vi "Get Bucket Location.vi"(8 "error in (no error)":errorcluster, 9 "Bucket":string) -> (0 "error out":errorcluster, 3 "Region":T1)   [LabVIEW 2015, in "LV Interface for Amazon S3.lvlib"]
doc: "This operation <B>returns</B> a <B>bucket's Region</B>. You set the bucket's Region using the Region request parameter in a PUT Bucket request. To use this implementation of the operation, <B>you must be the bucket Owner</B>."
uses:
  LV Interface for Amazon S3.lvlib
  Typedefs/AMZ_S3_LocationConstraint.ctl
  XML Parser/XML Parser.lvlib
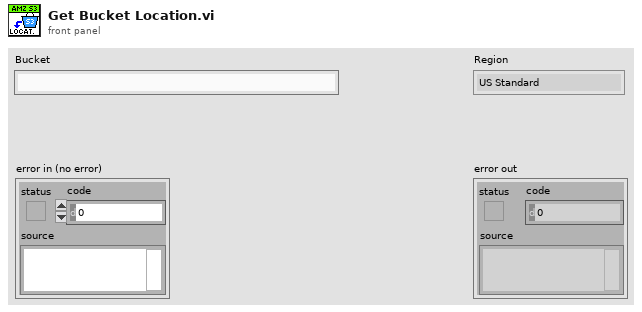
[diagram p1: front panel]
types:
  T1 = typedef "LV Interface for Amazon S3.lvlib/AMZ_S3_LocationConstraint.ctl" = enum16{"US Standard", "us-east-2", "us-west-1", "us-west-2", "ap-northeast-1", "ap-northeast-2", "ap-southeast-1", "ap-southeast-2", "ca-central-1", "eu-central-1", "eu-west-1", "eu-west-2", "sa-east-1"}
  T2 = typedef "LV Interface for Amazon S3.lvlib/AMZ_S3_Call Results.ctl" = enum16{"Success", "UndefinedError", "AccessDenied", "AccountProblem", "AmbiguousGrantByEmailAddress", "BadDigest", "BucketAlreadyExists", "BucketAlreadyOwnedByYou", "BucketNotEmpty", "CredentialsNotSupported", "CrossLocationLoggingProhibited", "EntityTooSmall", "EntityTooLarge", "ExpiredToken", "IllegalVersioningConfigurationException", "IncompleteBody", "IncorrectNumberOfFilesInPostRequest", "InlineDataTooLarge", "InternalError", "InvalidAccessKeyId", "InvalidAddressingHeader", "InvalidArgument", "InvalidBucketName", "InvalidDigest", "InvalidLocationConstraint", "InvalidPart", "InvalidPartOrder", "InvalidPayer", "InvalidPolicyDocument", "InvalidRange", "InvalidSecurity", "InvalidSOAPRequest", "InvalidStorageClass", "InvalidTargetBucketForLogging", "InvalidToken", "InvalidURI", "KeyTooLong", "MalformedACLError", "MalformedPOSTRequest", "MalformedXML", "MaxMessageLengthExceeded", "MaxPostPreDataLengthExceededError", "MetadataTooLarge", "MethodNotAllowed", "MissingAttachment", "MissingContentLength", "MissingRequestBodyError", "MissingSecurityElement", "MissingSecurityHeader", "NoLoggingStatusForKey", "NoSuchBucket", "NoSuchKey", "NoSuchUpload", "NoSuchVersion", "NotImplemented", "NotSignedUp", "OperationAborted", "PermanentRedirect", "PreconditionFailed", "Redirect", "RequestIsNotMultiPartContent", "RequestTimeout", "RequestTimeTooSkewed", "RequestTorrentOfBucketError", "SignatureDoesNotMatch", "SlowDown", "TemporaryRedirect", "TokenRefreshRequired", "TooManyBuckets", "UnexpectedContent", "UnresolvableGrantByEmailAddress", "UserKeyMustBeSpecified", "LabVIEWError"}
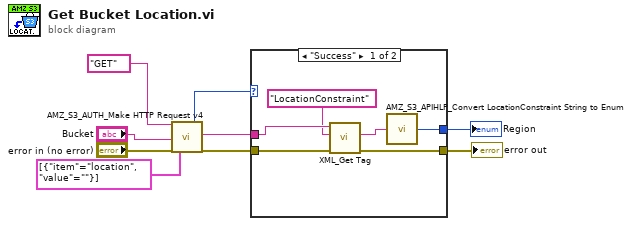
[diagram p0: block diagram]
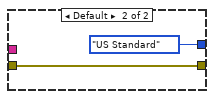
[diagram p2: hidden frame]
diagram:
  n1 = call "AMZ_S3_AUTH_Make HTTP Request v4.vi"("HTTP-Verb"="GET", "Bucket"="Bucket", "error in"="error in (no error)", "request parameters"=cluster{"item":string, "value":string}[] [{"item"="location", "value"=""}]) -> ("Call Result"=w2:T2, "response body"=w3:string, "error out"=w7:errorcluster)  [unwired: 12 in, 1 out]
  n2 = case shown="\"Success\"" w2 {
    tunnel: w7 -> [w15 w17]
    tunnel: w3 -> [w14 _]
    tunnel: [w12 w17] -> w9
    tunnel: [w10 AMZ_S3_LocationConstraint."US Standard" ("Location")] -> w8
    frame "Success" {
      n3 = call "XML_Get Tag.vi"("error in (no error)"=w15, "Tag name"="LocationConstraint", "XML String in"=w14) -> ("error out"=w12:errorcluster, "Tag value"=w11:string)  [unwired: 4 in, 3 out]
      n4 = call "AMZ_S3_APIHLP_Convert LocationConstraint String to Enum.vi"("Location String"=w11) -> ("Location"=w10:T1)  [unwired: 4 in]
    }
    frame Default {
    }
  }
  "error out" <- w9
  "Region" <- w8
